vi "Begin.vi"(8 "error in":errorcluster) -> (0 "error out":errorcluster)   [LabVIEW 2017]
doc: "Called before other user functions, this VI is expected to open initial I/O refnums, load in file data, and do all program initialization. Notice that the <B>error out</B> terminal is simply used for data flow. Wiring it to other structures or subVIs ensures that this VI runs first."
uses:
  <vilib>/Rock Robotics/WPI/DriverStation/WPI_DriverStationRobotMode2.ctl
  <vilib>/Rock Robotics/WPI/Joystick/WPI_JoystickDeviceEnum.ctl
  <vilib>/Rock Robotics/SystemInterfaces/DIO/FPGA_DIOPWMChannel.ctl
  <vilib>/Rock Robotics/SystemInterfaces/DIO/FPGA_DIOChannel.ctl
  <vilib>/Rock Robotics/WPI/Solenoid/WPI_SolenoidChannel.ctl
  <vilib>/Rock Robotics/WPI/ThirdParty/Phoenix-LabVIEW/Motor Controller/Controls/CTRE_Phoenix_MotorControl_NeutralMode.ctl
  <vilib>/Rock Robotics/WPI/ThirdParty/Phoenix-LabVIEW/Motor Controller/Controls/CTRE_Phoenix_MotorControl_LimitSwitchNormal.ctl
  <vilib>/Rock Robotics/WPI/ThirdParty/Phoenix-LabVIEW/Motor Controller/Controls/CTRE_Phoenix_MotorControl_LimitSwitchSource_Local.ctl
  Robot Global Data.vi
  <vilib>/Rock Robotics/WPI/Switch/WPI_SwitchOpenLimit.vi
  <vilib>/Rock Robotics/WPI/Solenoid/WPI_SolenoidOpenSingle.vi
  <vilib>/Rock Robotics/WPI/Counter/WPI_CounterDigitalInputToDigitalSource.vi
  <vilib>/Rock Robotics/WPI/MotorControl/WPI_MotorControlOpen VictorSP.vi
  Public/Documents/Cross The Road Electronics/Phoenix-LabVIEW/Motor Controller/Get/CTRE_Phoenix_MotorController_GetPulseWidthAll.vi
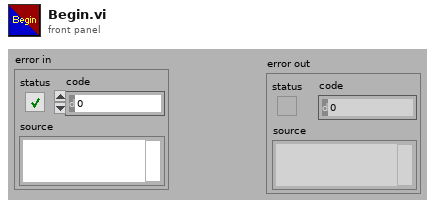
[diagram p1: front panel]
types:
  T1 = typedef "CTRE_Phoenix_MotorControl_LimitSwitchSource_Local.ctl" = enum16{"Feedback Connector", "Remote Talon SRX", "Remote CANifier", "Deactivated"}
  T2 = typedef "CTRE_Phoenix_MotorControl_LimitSwitchNormal.ctl" = enum16{"Normally Open", "Normally Closed", "Disabled"}
  T3 = typedef "CTRE_Phoenix_MotorControl_NeutralMode.ctl" = enum8{"EEPROMSetting", "Override to Coast", "Override to Brake"}
  T4 = typedef "FPGA_DIOPWMChannel.ctl" = enum8{"PWM 0", "PWM 1", "PWM 2", "PWM 3", "PWM 4", "PWM 5", "PWM 6", "PWM 7", "PWM 8", "PWM 9", "PWM MXP 0", "PWM MXP 1", "PWM MXP 2", "PWM MXP 3", "PWM MXP 4", "PWM MXP 5", "PWM MXP 6", "PWM MXP 7", "PWM MXP 8", "PWM MXP 9", "Invalid"}
  T5 = typedef "WPI_JoystickDeviceEnum.ctl" = enum16{"USB 0", "USB 1", "USB 2", "USB 3", "USB 4", "USB 5"}
  T6 = typedef "FPGA_DIOChannel.ctl" = enum8{"DIO 0", "DIO 1", "DIO 2", "DIO 3", "DIO 4", "DIO 5", "DIO 6", "DIO 7", "DIO 8", "DIO 9", "DIO MXP 0", "DIO MXP 1", "DIO MXP 2", "DIO MXP 3", "DIO MXP 4", "DIO MXP 5", "DIO MXP 6", "DIO MXP 7", "DIO MXP 8", "DIO MXP 9", "DIO MXP 10", "DIO MXP 11", "DIO MXP 12", "DIO MXP 13", "DIO MXP 14", "DIO MXP 15", "SPI Port CS1", "SPI Port CS2", "SPI Port CS3", "SPI Port MISO", "SPI Port MOSI", "Invalid"}
  T7 = typedef "WPI_SolenoidChannel.ctl" = enum8{"Solenoid 0", "Solenoid 1", "Solenoid 2", "Solenoid 3", "Solenoid 4", "Solenoid 5", "Solenoid 6", "Solenoid 7", "Invalid"}
  T8 = typedef "WPI_DriverStationRobotMode2.ctl" = enum16{"Autonomous Disabled", "Autonomous Enabled", "Teleop Disabled", "Teleop Enabled", "Disconnected", "Finish", "Test Disabled", "Test Enabled", "Emergency Stopped"}
  T9 = typedef "WPI_MotorControlDeviceRef.ctl" = cluster{"DeviceStatus":errorcluster, "Type":T10, "PWM":cluster{"PWM Channel":T4, "DeadBand":T11}, "CAN":cluster{"Device Number":u8, "SetOutput VI Ref":variant, "GetOutput VI Ref":variant, "Enable VI Ref":variant, "Disable VI Ref":variant, "Data":variant}, "Invert":bool, "DIO PWM":cluster{"PWM \"Enable\" Channel":T4, "DIOChannel":T6, "PWM Rate":dbl}}
  T10 = typedef "WPI_MotorControlType.ctl" = enum16{"PWM", "CAN", "DIO PWM"}
  T11 = typedef "WPI_PWMDeadband.ctl" = cluster{"Name":string, "maxPositivePwm":i32, "minPositivePwm":i32, "centerPwm":i32, "maxNegativePwm":i32, "minNegativePwm":i32, "angularRange":u16}
  T12 = typedef "WPI_ServoDeviceRef.ctl" = cluster{"DeviceStatus":errorcluster, "PWM Channel":T4, "DeadBand":T11}
  T13 = typedef "WPI_DigitalInputDevRef.ctl" = cluster{"DevStatus":errorcluster, "DIO Channel":T6}
  T14 = typedef "FPGA_CounterEncoderSourceConvertionLVSourceType.ctl" = cluster{"DevStatus":errorcluster, "AnalogTriggerMode?":bool, "DigitalMode":cluster{"DIO Channel":T15}, "AnalogTriggerMode":cluster{"AnalogTriggerIndex":T16, "OutputType":T17}}
  T15 = typedef "FPGA_DIODigitalSourceChannel.ctl" = enum8{"DIO 0", "DIO 1", "DIO 2", "DIO 3", "DIO 4", "DIO 5", "DIO 6", "DIO 7", "DIO 8", "DIO 9", "DIO MXP 0", "DIO MXP 1", "DIO MXP 2", "DIO MXP 3", "DIO MXP 4", "DIO MXP 5", "DIO MXP 6", "DIO MXP 7", "DIO MXP 8", "DIO MXP 9", "DIO MXP 10", "DIO MXP 11", "DIO MXP 12", "DIO MXP 13", "DIO MXP 14", "DIO MXP 15", "Disabled"}
  T16 = typedef "FPGA_AnalogTriggerIndex.ctl" = enum8{"Trig 0", "Trig 1", "Trig 2", "Trig 3", "Trig 4", "Trig 5", "Trig 6", "Trig 7", "Invalid"}
  T17 = typedef "FPGA_AnalogTriggerOutType.ctl" = enum16{"InWindow", "TriggerState", "Rising", "Falling"}
  T18 = typedef "WPI_EncoderDevRef.ctl" = cluster{"DevStatus":errorcluster, "EncoderIndex":T19, "CounterIndex":T20, "DistancePerCount":dbl, "Decoding Type":T21}
  T19 = typedef "FPGA_EncoderIdx.ctl" = enum8{"Enc 0", "Enc 1", "Enc 2", "Enc 3", "Enc 4", "Enc 5", "Enc 6", "Enc 7", "Invalid"}
  T20 = typedef "FPGA_CounterCtrSystemIndex.ctl" = enum8{"Ctr 0", "Ctr 1", "Ctr 2", "Ctr 3", "Ctr 4", "Ctr 5", "Ctr 6", "Ctr 7", "Invalid"}
  T21 = typedef "WPI_EncoderType.ctl" = enum16{"1x", "2x", "4x"}
  T22 = typedef "WPI_SolenoidDevRef.ctl" = cluster{"DevStatus":errorcluster, "Pneumatics Control Module":u8, "Forward Solenoid Channel":T7, "Reverse Solenoid Channel":T7}
  T23 = typedef "WPI_JoystickDevRef.ctl" = cluster{"Device":T5}
  T24 = typedef "WPI_SwitchDevRef.ctl" = cluster{"DevStatus":errorcluster, "DIO Channel":T6, "CntIndex":T20, "Normally Closed":bool}
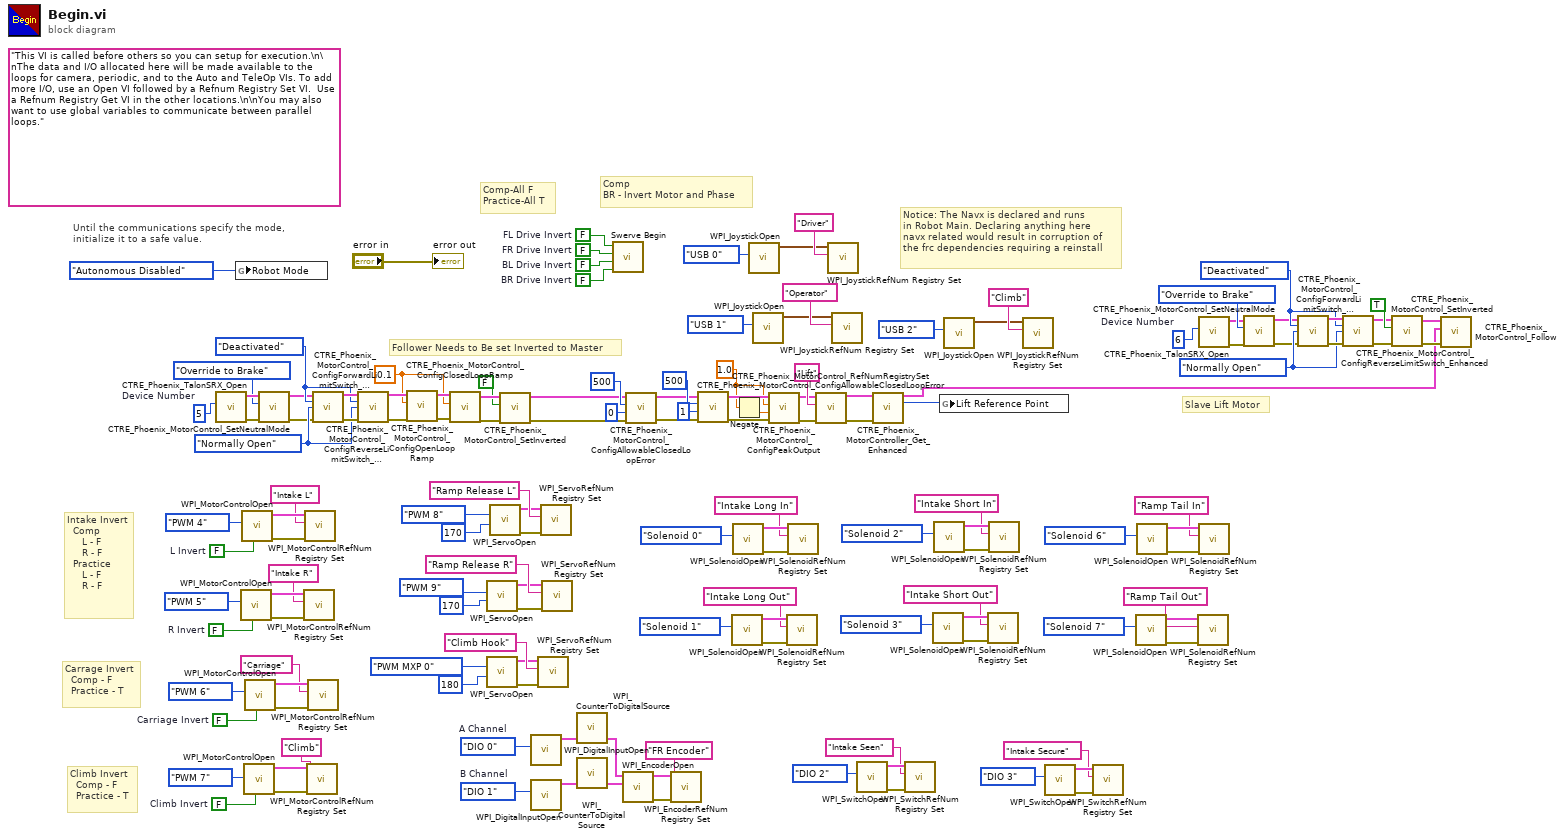
[diagram p0: block diagram]
diagram:
  w13 = CTRE_Phoenix_MotorControl_LimitSwitchSource_Local."Deactivated" ("Limit Switch Source")
  w14 = CTRE_Phoenix_MotorControl_LimitSwitchNormal."Normally Open" ("NormallyOpenOrClosed")
  w18 = u8 6  # Device Number
  w19 = FALSE  # Climb Invert
  w24 = 1.0 ("x")
  w30 = FALSE  # Carriage Invert
  w31 = FALSE  # R Invert
  w32 = FALSE  # L Invert
  w37 = FALSE  # FL Drive Invert
  w38 = FALSE  # FR Drive Invert
  w39 = FALSE  # BL Drive Invert
  w40 = FALSE  # BR Drive Invert
  w84 = FPGA_DIOChannel."DIO 1"  # B Channel
  w83 = FPGA_DIOChannel."DIO 0"  # A Channel
  w85 = CTRE_Phoenix_MotorControl_LimitSwitchSource_Local."Deactivated" ("Limit Switch Source")
  w122 = u8 5  # Device Number
  w73 = 0.1 ("secondsFromNeutralToFull")
  w126 = CTRE_Phoenix_MotorControl_LimitSwitchNormal."Normally Open" ("NormallyOpenOrClosed")
  (unwired) "This VI is called before others so you can setup for execution.\n\nThe data and I/O allocated here will be made available to the loops for camera, periodic, and to the Auto and TeleOp VIs. To add more I/O, use an Open VI followed by a Refnum Registry Set VI.  Use a Refnum Registry Get VI in the other locations.\n\nYou may also want to use global variables to communicate between parallel loops."
  # "Slave Lift Motor"
  # "Notice: The Navx is declared and runs\nin Robot Main. Declaring anything here\nnavx related would result in corruption of\nthe frc dependencies requiring a reinstall"
  # "Follower Needs to Be set Inverted to Master"
  # "Comp\nBR - Invert Motor and Phase"
  # "Climb Invert\n  Comp - F\n  Practice - T"
  # "Carrage Invert\n  Comp - F\n  Practice - T"
  # "Intake Invert\n  Comp\n     L - F\n     R - F\n  Practice\n     L - F\n     R - F"
  # "Comp-All F\nPractice-All T"
  # "Until the communications specify the mode,\ninitialize it to a safe value."
  n1 = call <vilib>:"CTRE_Phoenix_TalonSRX_Open.vi"("Device Number"=w122) -> ("error out"=w131:errorcluster, "CAN Talon SRX Ref"=w130:T9)  [unwired: 9 in]
  n2 = global write "Robot Global Data.vi" "Robot Mode"(WPI_DriverStationRobotMode2."Autonomous Disabled" ("Robot Mode")) -> ()
  n3 = call-poly <vilib>:"WPI_MotorControlOpen.vi"("Invert"=w31, "PWM Channel"=FPGA_DIOPWMChannel."PWM 5") -> ("error out"=w36:errorcluster, "MotorControlDeviceRef"=w35:T9)  [unwired: 8 in]
  n4 = call-poly <vilib>:"WPI_MotorControlOpen.vi"("Invert"=w32, "PWM Channel"=FPGA_DIOPWMChannel."PWM 4") -> ("error out"=w135:errorcluster, "MotorControlDeviceRef"=w134:T9)  [unwired: 8 in]
  n5 = call-poly <vilib>:"WPI_MotorControlOpen.vi"("Invert"=w19, "PWM Channel"=FPGA_DIOPWMChannel."PWM 7") -> ("error out"=w121:errorcluster, "MotorControlDeviceRef"=w120:T9)  [unwired: 8 in]
  n6 = call-poly <vilib>:"WPI_MotorControlOpen.vi"("Invert"=w30, "PWM Channel"=FPGA_DIOPWMChannel."PWM 6") -> ("error out"=w72:errorcluster, "MotorControlDeviceRef"=w71:T9)  [unwired: 8 in]
  n7 = call <vilib>:"CTRE_Phoenix_MotorControl_SetNeutralMode.vi"("error in (no error)"=w131, "Motor Control Neutral Mode"=CTRE_Phoenix_MotorControl_NeutralMode."Override to Brake", "PhoenixMotorControlDevRef"=w130) -> ("error out"=w52:errorcluster, "PhoenixMotorControlDevRef"=w53:T9)  [unwired: 7 in]
  n8 = call <vilib>:"WPI_MotorControlRefNum Registry Set.vi"("error in (no error)"=w36, "refnum name"="Intake R", "MotorControlDevRef"=w35) -> ()  [unwired: 7 in, 2 out]
  n9 = call <vilib>:"WPI_MotorControlRefNum Registry Set.vi"("error in (no error)"=w135, "refnum name"="Intake L", "MotorControlDevRef"=w134) -> ()  [unwired: 7 in, 2 out]
  n10 = call <vilib>:"WPI_MotorControlRefNum Registry Set.vi"("error in (no error)"=w121, "refnum name"="Climb", "MotorControlDevRef"=w120) -> ()  [unwired: 7 in, 2 out]
  n11 = call <vilib>:"WPI_MotorControlRefNum Registry Set.vi"("error in (no error)"=w72, "refnum name"="Carriage", "MotorControlDevRef"=w71) -> ()  [unwired: 7 in, 2 out]
  n12 = call <vilib>:"CTRE_Phoenix_MotorControl_ConfigForwardLimitSwitch_Enhanced.vi"("PhoenixMotorControlDevRef"=w53, "Limit Switch Source"=w85, "NormallyOpenOrClosed"=w126, "error in (no error)"=w52) -> ("PhoenixMotorControlDevRef"=w128:T9, "error out"=w127:errorcluster)  [unwired: 10 in]
  n13 = call <vilib>:"CTRE_Phoenix_MotorControl_ConfigReverseLimitSwitch_Enhanced.vi"("PhoenixMotorControlDevRef"=w128, "Limit Switch Source"=w85, "NormallyOpenOrClosed"=w126, "error in (no error)"=w127) -> ("PhoenixMotorControlDevRef"=w124:T9, "error out"=w125:errorcluster)  [unwired: 10 in]
  n14 = call <vilib>:"CTRE_Phoenix_MotorControl_ConfigOpenLoopRamp.vi"("error in (no error)"=w125, "secondsFromNeutralToFull"=w73, "PhoenixMotorControlDevRef"=w124) -> ("error out"=w75:errorcluster, "PhoenixMotorControlDevRef"=w74:T9)  [unwired: 7 in]
  n15 = call <vilib>:"CTRE_Phoenix_MotorControl_ConfigClosedLoopRamp.vi"("error in (no error)"=w75, "secondsFromNeutralToFull"=w73, "PhoenixMotorControlDevRef"=w74) -> ("error out"=w50:errorcluster, "PhoenixMotorControlDevRef"=w51:T9)  [unwired: 7 in]
  n16 = call <vilib>:"WPI_ServoOpen.vi"("Angular Range"=u16 170, "PWM Channel"=FPGA_DIOPWMChannel."PWM 9") -> ("error out"=w64:errorcluster, "ServoDeviceRef"=w63:T12)  [unwired: 8 in]
  n17 = call <vilib>:"WPI_ServoOpen.vi"("Angular Range"=u16 180, "PWM Channel"=FPGA_DIOPWMChannel."PWM MXP 0") -> ("error out"=w57:errorcluster, "ServoDeviceRef"=w56:T12)  [unwired: 8 in]
  n18 = call <vilib>:"WPI_ServoOpen.vi"("Angular Range"=u16 170, "PWM Channel"=FPGA_DIOPWMChannel."PWM 8") -> ("error out"=w66:errorcluster, "ServoDeviceRef"=w65:T12)  [unwired: 8 in]
  n19 = call <vilib>:"CTRE_Phoenix_MotorControl_SetInverted.vi"("error in (no error)"=w50, "Invert?"=FALSE, "PhoenixMotorControlDevRef"=w51) -> ("error out"=w1:errorcluster, "PhoenixMotorControlDevRef"=w2:T9)  [unwired: 7 in]
  n20 = call <vilib>:"WPI_DigitalInputOpen.vi"("DIO Channel"=w83) -> ("DigitalInputDevRef"=w80:T13)  [unwired: 1 in, 9 out]
  n21 = call <vilib>:"WPI_DigitalInputOpen.vi"("DIO Channel"=w84) -> ("DigitalInputDevRef"=w81:T13)  [unwired: 1 in, 9 out]
  n22 = call <vilib>:"WPI_ServoRefNum Registry Set.vi"("error in (no error)"=w57, "refnum name"="Climb Hook", "ServoDeviceRef"=w56) -> ()  [unwired: 7 in, 2 out]
  n23 = call <vilib>:"WPI_ServoRefNum Registry Set.vi"("error in (no error)"=w66, "refnum name"="Ramp Release L", "ServoDeviceRef"=w65) -> ()  [unwired: 7 in, 2 out]
  n24 = call <vilib>:"WPI_ServoRefNum Registry Set.vi"("error in (no error)"=w64, "refnum name"="Ramp Release R", "ServoDeviceRef"=w63) -> ()  [unwired: 7 in, 2 out]
  n25 = call-poly <vilib>:"WPI_CounterToDigitalSource.vi"("DigitalInputDevRef"=w80) -> ("Digital Source"=w79:T14)  [unwired: 6 out]
  n26 = call-poly <vilib>:"WPI_CounterToDigitalSource.vi"("DigitalInputDevRef"=w81) -> ("Digital Source"=w82:T14)  [unwired: 6 out]
  n27 = call "Swerve Begin.vi"("BR Drive Invert"=w40, "BL Drive Invert"=w39, "FR Drive Invert"=w38, "FL Drive Invert"=w37) -> ()  [unwired: 8 in]
  n28 = call <vilib>:"WPI_EncoderOpen.vi"("BSource"=w82, "ASource"=w79) -> ("error out"=w78:errorcluster, "EncoderDevRef"=w77:T18)  [unwired: 6 in, 2 out]
  n29 = call <vilib>:"CTRE_Phoenix_MotorControl_ConfigAllowableClosedLoopError.vi"("error in (no error)"=w1, "slotIdx"=u32 0, "allowableClosedLoopError"=500, "PhoenixMotorControlDevRef"=w2) -> ("error out"=w21:errorcluster, "PhoenixMotorControlDevRef"=w20:T9)  [unwired: 6 in]
  n30 = call <vilib>:"WPI_EncoderRefNum Registry Set.vi"("error in (no error)"=w78, "refnum name"="FR Encoder", "EncoderDevRef"=w77) -> ()  [unwired: 7 in, 2 out]
  n31 = call <vilib>:"CTRE_Phoenix_MotorControl_ConfigAllowableClosedLoopError.vi"("error in (no error)"=w21, "slotIdx"=u32 1, "allowableClosedLoopError"=500, "PhoenixMotorControlDevRef"=w20) -> ("error out"=w28:errorcluster, "PhoenixMotorControlDevRef"=w29:T9)  [unwired: 6 in]
  n32 = call-poly <vilib>:"WPI_SolenoidOpen.vi"("Solenoid Channel"=WPI_SolenoidChannel."Solenoid 1") -> ("error out"=w96:errorcluster, "SolenoidDevRef"=w95:T22)  [unwired: 9 in]
  n33 = call-poly <vilib>:"WPI_SolenoidOpen.vi"("Solenoid Channel"=WPI_SolenoidChannel."Solenoid 0") -> ("error out"=w100:errorcluster, "SolenoidDevRef"=w99:T22)  [unwired: 9 in]
  n34 = Negate(x=w24) -> (-x=w25:dbl)
  n35 = call <vilib>:"WPI_JoystickOpen.vi"("JoystickDevice"=WPI_JoystickDeviceEnum."USB 0") -> ("JoystickDevRef"=w141:T23)  [unwired: 10 in]
  n36 = call <vilib>:"WPI_JoystickOpen.vi"("JoystickDevice"=WPI_JoystickDeviceEnum."USB 1") -> ("JoystickDevRef"=w137:T23)  [unwired: 10 in]
  n37 = call <vilib>:"CTRE_Phoenix_MotorControl_ConfigPeakOutput.vi"("error in (no error)"=w28, "Reverse Peak Percent Output"=w25, "Forward Peak Percent Output"=w24, "PhoenixMotorControlDevRef"=w29) -> ("error out"=w26:errorcluster, "PhoenixMotorControlDevRef"=w27:T9)  [unwired: 6 in]
  n38 = call <vilib>:"WPI_SolenoidRefNum Registry Set.vi"("error in (no error)"=w96, "refnum name"="Intake Long Out", "SolenoidDevRef"=w95) -> ()  [unwired: 7 in, 2 out]
  n39 = call <vilib>:"WPI_SolenoidRefNum Registry Set.vi"("error in (no error)"=w100, "refnum name"="Intake Long In", "SolenoidDevRef"=w99) -> ()  [unwired: 7 in, 2 out]
  n40 = call <vilib>:"CTRE_Phoenix_MotorControl_RefNumRegistrySet.vi"("error in (no error)"=w26, "refnum name"="Lift", "PhoenixMotorControlDevRef"=w27) -> ("error out"=w42:errorcluster, "PhoenixMotorControlDevRef"=w43:T9)  [unwired: 7 in]
  n41 = call <vilib>:"WPI_JoystickRefNum Registry Set.vi"("refnum name"="Driver", "JoystickDevRef"=w141) -> ()  [unwired: 8 in, 2 out]
  n42 = call <vilib>:"WPI_JoystickRefNum Registry Set.vi"("refnum name"="Operator", "JoystickDevRef"=w137) -> ()  [unwired: 8 in, 2 out]
  n43 = call-poly <vilib>:"WPI_SwitchOpen.vi"("DIO Channel"=FPGA_DIOChannel."DIO 2") -> ("error out"=w117:errorcluster, "SwitchDevRef"=w116:T24)  [unwired: 9 in]
  n44 = call-poly "CTRE_Phoenix_MotorController_Get_Enhanced.vi"("PhoenixMotorControlDevRef"=w43, "error in"=w42) -> ("PhoenixMotorControlDevRef"=w3:T9, "Pulse Width Position"=w41:i32)  [unwired: 8 in, 4 out]
  n45 = call <vilib>:"WPI_SwitchRefNum Registry Set.vi"("error in (no error)"=w117, "refnum name"="Intake Seen", "SwitchDevRef"=w116) -> ()  [unwired: 7 in, 2 out]
  n46 = call-poly <vilib>:"WPI_SolenoidOpen.vi"("Solenoid Channel"=WPI_SolenoidChannel."Solenoid 3") -> ("error out"=w88:errorcluster, "SolenoidDevRef"=w87:T22)  [unwired: 9 in]
  n47 = call-poly <vilib>:"WPI_SolenoidOpen.vi"("Solenoid Channel"=WPI_SolenoidChannel."Solenoid 2") -> ("error out"=w92:errorcluster, "SolenoidDevRef"=w91:T22)  [unwired: 9 in]
  n48 = global write "Robot Global Data.vi" "Lift Reference Point"(w41) -> ()
  n49 = call <vilib>:"WPI_JoystickOpen.vi"("JoystickDevice"=WPI_JoystickDeviceEnum."USB 2") -> ("JoystickDevRef"=w45:T23)  [unwired: 10 in]
  n50 = call <vilib>:"WPI_SolenoidRefNum Registry Set.vi"("error in (no error)"=w88, "refnum name"="Intake Short Out", "SolenoidDevRef"=w87) -> ()  [unwired: 7 in, 2 out]
  n51 = call <vilib>:"WPI_SolenoidRefNum Registry Set.vi"("error in (no error)"=w92, "refnum name"="Intake Short In", "SolenoidDevRef"=w91) -> ()  [unwired: 7 in, 2 out]
  n52 = call <vilib>:"WPI_JoystickRefNum Registry Set.vi"("refnum name"="Climb", "JoystickDevRef"=w45) -> ()  [unwired: 8 in, 2 out]
  n53 = call-poly <vilib>:"WPI_SwitchOpen.vi"("DIO Channel"=FPGA_DIOChannel."DIO 3") -> ("error out"=w113:errorcluster, "SwitchDevRef"=w112:T24)  [unwired: 9 in]
  n54 = call <vilib>:"WPI_SwitchRefNum Registry Set.vi"("error in (no error)"=w113, "refnum name"="Intake Secure", "SwitchDevRef"=w112) -> ()  [unwired: 7 in, 2 out]
  n55 = call-poly <vilib>:"WPI_SolenoidOpen.vi"("Solenoid Channel"=WPI_SolenoidChannel."Solenoid 7") -> ("error out"=w104:errorcluster, "SolenoidDevRef"=w103:T22)  [unwired: 9 in]
  n56 = call-poly <vilib>:"WPI_SolenoidOpen.vi"("Solenoid Channel"=WPI_SolenoidChannel."Solenoid 6") -> ("error out"=w108:errorcluster, "SolenoidDevRef"=w107:T22)  [unwired: 9 in]
  n57 = call <vilib>:"WPI_SolenoidRefNum Registry Set.vi"("error in (no error)"=w104, "refnum name"="Ramp Tail Out", "SolenoidDevRef"=w103) -> ()  [unwired: 7 in, 2 out]
  n58 = call <vilib>:"CTRE_Phoenix_TalonSRX_Open.vi"("Device Number"=w18) -> ("error out"=w9:errorcluster, "CAN Talon SRX Ref"=w10:T9)  [unwired: 9 in]
  n59 = call <vilib>:"WPI_SolenoidRefNum Registry Set.vi"("error in (no error)"=w108, "refnum name"="Ramp Tail In", "SolenoidDevRef"=w107) -> ()  [unwired: 7 in, 2 out]
  n60 = call <vilib>:"CTRE_Phoenix_MotorControl_SetNeutralMode.vi"("error in (no error)"=w9, "Motor Control Neutral Mode"=CTRE_Phoenix_MotorControl_NeutralMode."Override to Brake", "PhoenixMotorControlDevRef"=w10) -> ("error out"=w11:errorcluster, "PhoenixMotorControlDevRef"=w12:T9)  [unwired: 7 in]
  n61 = call <vilib>:"CTRE_Phoenix_MotorControl_ConfigForwardLimitSwitch_Enhanced.vi"("PhoenixMotorControlDevRef"=w12, "Limit Switch Source"=w13, "NormallyOpenOrClosed"=w14, "error in (no error)"=w11) -> ("PhoenixMotorControlDevRef"=w16:T9, "error out"=w15:errorcluster)  [unwired: 10 in]
  n62 = call <vilib>:"CTRE_Phoenix_MotorControl_ConfigReverseLimitSwitch_Enhanced.vi"("PhoenixMotorControlDevRef"=w16, "Limit Switch Source"=w13, "NormallyOpenOrClosed"=w14, "error in (no error)"=w15) -> ("PhoenixMotorControlDevRef"=w7:T9, "error out"=w6:errorcluster)  [unwired: 10 in]
  n63 = call <vilib>:"CTRE_Phoenix_MotorControl_SetInverted.vi"("error in (no error)"=w6, "Invert?"=TRUE, "PhoenixMotorControlDevRef"=w7) -> ("error out"=w4:errorcluster, "PhoenixMotorControlDevRef"=w5:T9)  [unwired: 7 in]
  n64 = call <vilib>:"CTRE_Phoenix_MotorControl_Follow.vi"("error in (no error)"=w4, "Master Controller to Follow"=w3, "PhoenixMotorControlDevRef"=w5) -> ()  [unwired: 7 in, 2 out]
  "error out" <- "error in"
